vi "luna_read.vi"() -> ()   [LabVIEW 2012]
uses:
  <vilib>/LabVIEW Interface for Arduino/Type Defs/Connection Type.ctl
  <vilib>/LabVIEW Interface for Arduino/Type Defs/Board Type.ctl
panel:
  out "decimal integer string":string
  in  "stop 2":bool
  out "error out":errorcluster
  in  "error in (no error)":errorcluster
  in  "error in":errorcluster
  in  "Connection Type (USB/Serial)":T1
  in  "Bytes Per Packet (15)":u32=15
  in  "Board Type (Uno)":T2
  in  "Baud Rate (115200)":u32=115200
  in  "VISA resource":refnum<visa-resource-name>
  out "Error Out 2":errorcluster
  out "String 4":string
  in  "stop":bool
  out "data out":string
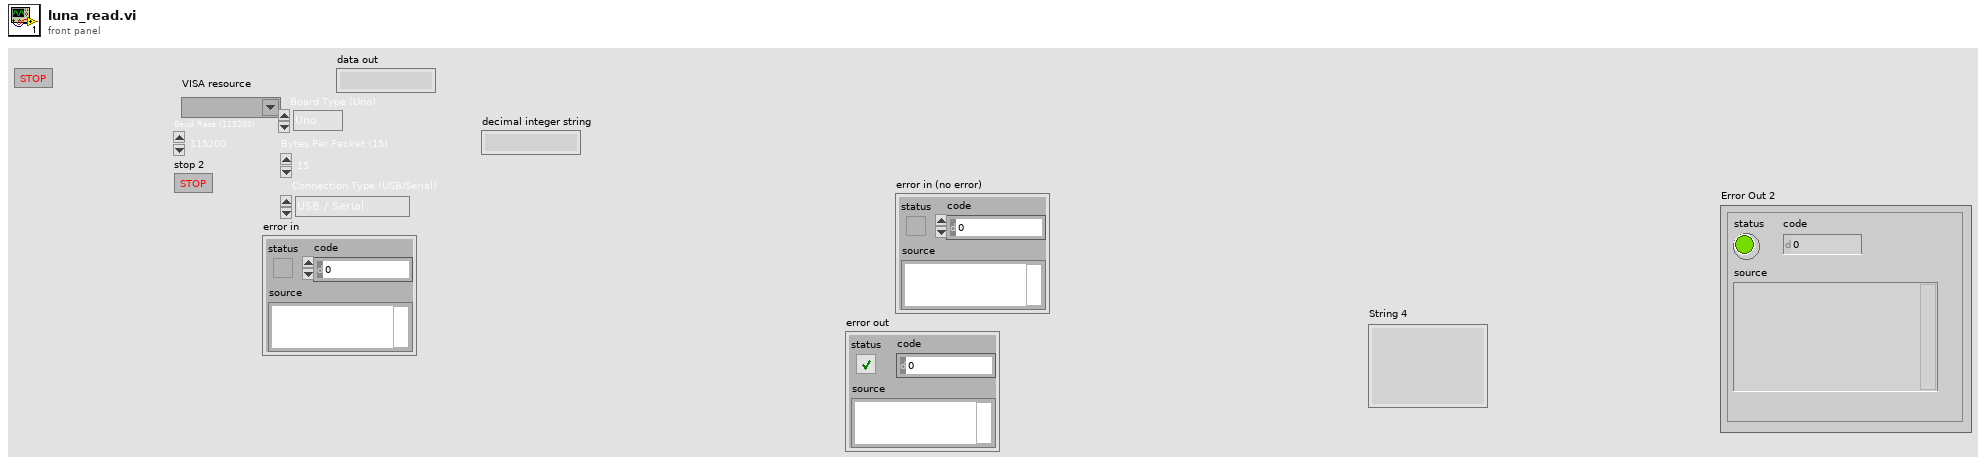
[diagram p1: front panel]
types:
  T1 = typedef "LabVIEW Interface for Arduino.lvlib/Connection Type.ctl" = enum8{"USB / Serial", "XBEE", "BlueSmirf (Bluetooth)"}
  T2 = typedef "LabVIEW Interface for Arduino.lvlib/Board Type.ctl" = enum16{"Uno", "Dimuelanove w/Atmega 328", "Mega 2560"}
  T3 = typedef "LabVIEW Interface for Arduino.lvlib/Arduino Resource.ctl" = cluster{"VISA resource":refnum<visa-resource-name>, "Board Type":T2, "Connection Type":enum8{"USB / Serial"}, "Bytes Per Packet (15)":u8}
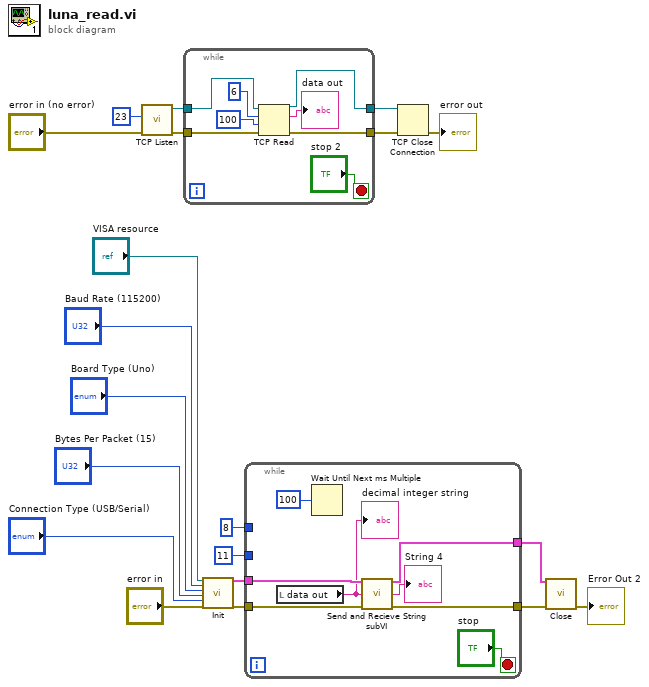
[diagram p0: block diagram]
diagram:
  n1 = call <vilib>:"TCP Listen.vi"("error in (no error)"="error in (no error)", "port"=u16 23) -> ("error out"=w2:errorcluster, "connection ID"=w5:refnum<k5>)  [unwired: 5 in, 3 out]
  n2 = while {
    tunnel: w5 -> [w26]
    tunnel: [w25] -> w4
    tunnel: [w24] -> w3
    tunnel: w2 -> [w23]
    stop <- "stop 2" stop-if-true
    n3 = TCP Read(connection ID=w26, bytes to read=6, error in (no error)=w23, 9:100 ("timeout ms (25000)")) -> (connection ID out=w25:refnum<k5>, data out=→"data out":string, error out=w24:errorcluster)  [unwired: 1 in]
  }
  n4 = call <vilib>:"Init.vi"("VISA resource"="VISA resource", "Baud Rate (115200)"="Baud Rate (115200)", "Board Type (Uno)"="Board Type (Uno)", "Bytes Per Packet (15)"="Bytes Per Packet (15)", "Connection Type (USB/Serial)"="Connection Type (USB/Serial)", "error in"="error in") -> ("Arduino Resource"=w20:T3, "error out"=w19:errorcluster)  [unwired: 12 in]
  n5 = while {
    tunnel: w20 -> [w33]
    tunnel: w19 -> [w32]
    tunnel: [w31] -> w17
    tunnel: [w30] -> w16
    tunnel: 11 -> [_]
    tunnel: 8 -> [_]
    stop <- "stop" stop-if-true
    n6 = local read "data out"() -> (w29:string)
    "decimal integer string" <- w29
    n7 = Wait Until Next ms Multiple(millisecond multiple=u32 100) -> ()  [unwired: 1 out]
    n8 = call "Send and Recieve String subVI.vi"("Arduino Resource"=w33, "String"=w29, "error in"=w32) -> ("Arduino Resource 2"=w31:T3, "String Output"=→"String 4":string, "error out"=w30:errorcluster)  [unwired: 10 in]
  }
  n9 = TCP Close Connection(connection ID=w4, error in (no error)=w3) -> (error out=→"error out":errorcluster)  [unwired: 1 in, 1 out]
  n10 = call <vilib>:"Close.vi"("Arduino Resource"=w17, "error in"=w16) -> ("error out"=→"Error Out 2":errorcluster)  [unwired: 13 in]
